vi "Autonics_Move.vi"(7 "Direction (+)":string="+", 8 "error in (no error)":errorcluster, 9 "Travel per Pulse (mm)":dbl=0.002, 10 "Move Distance (mm)":dbl=1.0, 11 "VISA resource name":refnum<visa-resource-name>) -> (0 "error out":errorcluster, 3 "VISA resource name out":refnum<visa-resource-name>)   [LabVIEW 2018]
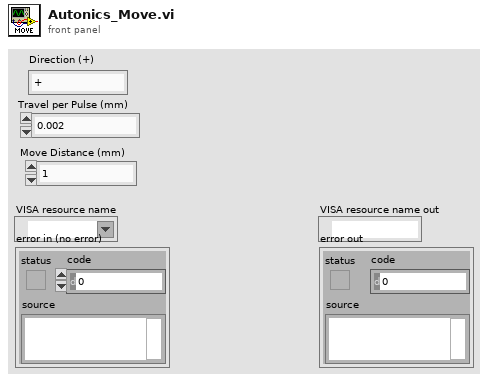
[diagram p1: front panel]
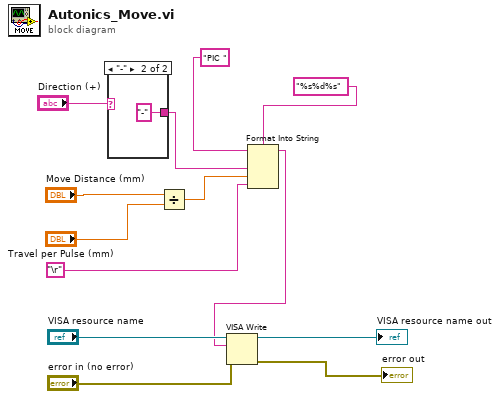
[diagram p0: block diagram]
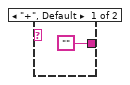
[diagram p2: hidden frame]
diagram:
  n1 = case shown="\"-\"" "Direction (+)" {
    tunnel: ["" "-"] -> w6
    frame "+", Default {
    }
    frame "-" {
    }
  }
  n2 = Divide(x="Move Distance (mm)", y="Travel per Pulse (mm)") -> (x/y=w9:dbl)
  n3 = Format Into String(format string="%s%d%s", initial string="PIC " ("string"), w6, w9, "\r") -> (resulting string=w1:string)  [unwired: 1 in, 1 out]
  n4 = VISA Write(VISA resource name="VISA resource name", write buffer=w1, error in (no error)="error in (no error)") -> (VISA resource name out=→"VISA resource name out":refnum<visa-resource-name>, error out=→"error out":errorcluster)  [unwired: 1 out]
